vi "RotationRun.vi"(11 "Data Cluster en entrée":T1) -> (2 "Booléen":bool, 3 "Data Cluster en sortie":T1)   [LabVIEW 2020]
uses:
  controls/UI Data.ctl
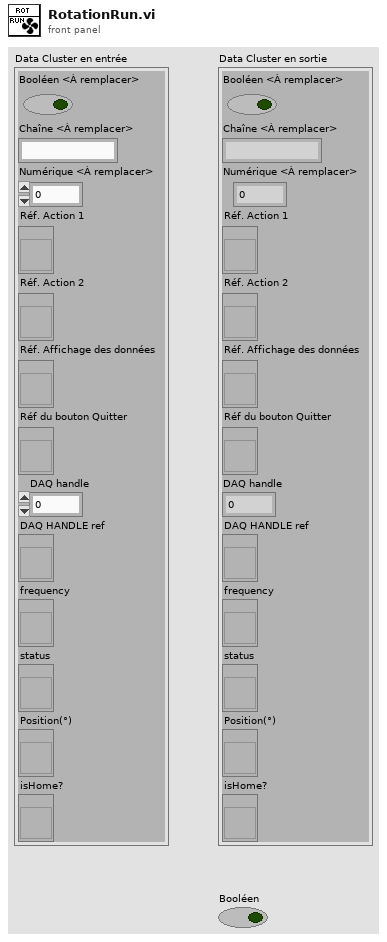
[diagram p1: front panel]
types:
  T1 = typedef "UI Data.ctl" = cluster{"Booléen <À remplacer>":bool, "Chaîne <À remplacer>":string, "Numérique <À remplacer>":dbl, "Réf. Action 1":refnum<vi>, "Réf. Action 2":refnum<vi>, "Réf. Affichage des données":refnum<vi>, "Réf du bouton Quitter":refnum<vi>, "DAQ handle":u32, "DAQ HANDLE ref":refnum<vi>, "frequency":refnum<vi>, "status":refnum<vi>, "Position(°)":refnum<vi>, "isHome?":refnum<vi>}
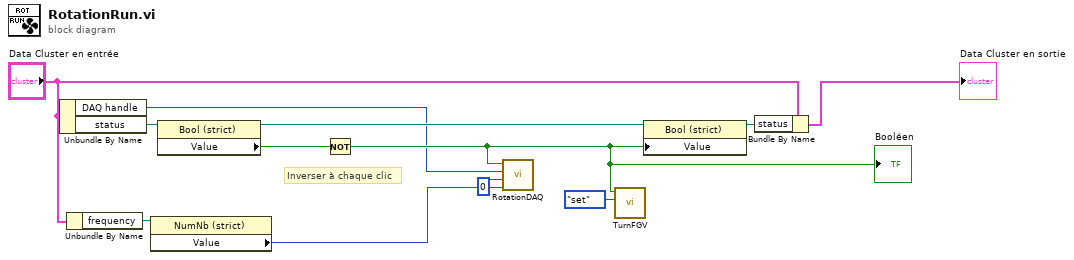
[diagram p0: block diagram]
diagram:
  # "Inverser à chaque clic"
  n1 = Unbundle By Name("Data Cluster en entrée") -> ("DAQ handle"=w2:u32, "status"=w8:refnum<vi>)
  n2 = Unbundle By Name("Data Cluster en entrée") -> ("frequency"=w10:refnum<vi>)
  n3 = property class="NumNb (strict)"(reference=w10) -> ("Value"=w9:i32)  [unwired: 1 in, 2 out]
  n4 = property class="Bool (strict)"(reference=w8) -> (reference out=w12:refnum<vi>, "Value"=w6:bool)  [unwired: 1 in, 1 out]
  n5 = Not(x=w6) -> (.not. x?=w7:bool)
  "Booléen" <- w7
  n6 = call "RotationDAQ.vi"("frequency"=w9, "pin"=0, "handle"=w2, "Tourner?"=w7) -> ()  [unwired: 7 in, 1 out]
  n7 = call "TurnFGV.vi"("Énum"=enum16{"set", "get"}."set", "set"=w7) -> ()  [unwired: 9 in, 1 out]
  n8 = property class="Bool (strict)"(reference=w12, "Value"=w7) -> (reference out=w5:refnum<vi>)  [unwired: 1 in, 1 out]
  n9 = Bundle By Name(cluster="Data Cluster en entrée", "status"=w5) -> (→"Data Cluster en sortie":T1)
